vi "TypeConv_Register Existing Namespaces.vi"(10 "Existing Module":refnum<vi>, 11 "Namespaces":T1[](array[typedef])) -> ()   [LabVIEW 2013]
uses:
  Data Structures/JSON/Namespace.ctl
  Data Structures/JSON/Enum.ctl
  Data Structures/JSON/Enum Value.ctl
  Data Structures/JSON/Method.ctl
  Data Structures/JSON/Param.ctl
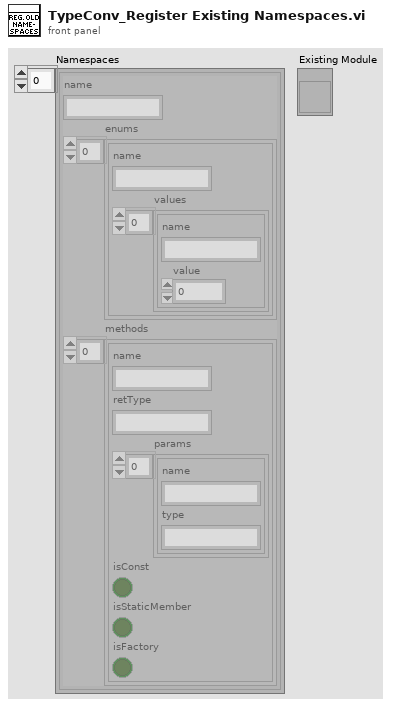
[diagram p1: front panel]
types:
  T1 = typedef "Namespace.ctl" = cluster{"name":string, "enums":T2[], "methods":T4[]}
  T2 = typedef "Enum.ctl" = cluster{"name":string, "values":T3[]}
  T3 = typedef "Enum Value.ctl" = cluster{"name":string, "value":i32}
  T4 = typedef "Method.ctl" = cluster{"name":string, "retType":string, "params":T5[], "isConst":bool, "isStaticMember":bool, "isFactory":bool}
  T5 = typedef "Param.ctl" = cluster{"name":string, "type":string}
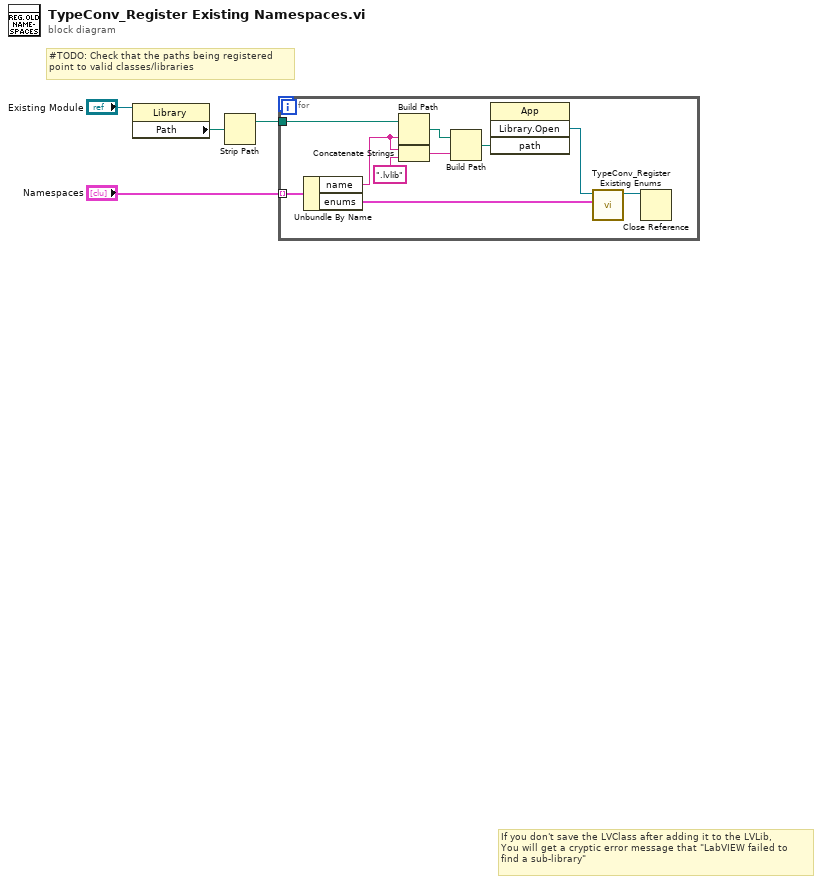
[diagram p0: block diagram]
diagram:
  # "#TODO: Check that the paths being registered\npoint to valid classes/libraries"
  # "If you don't save the LVClass after adding it to the LVLib,\nYou will get a cryptic error message that \"LabVIEW failed to\nfind a sub-library\""
  n1 = property class="Library"(reference="Existing Module") -> ("Path"=w2:path)  [unwired: 1 in, 2 out]
  n2 = Strip Path(path=w2) -> (stripped path=w1:path)  [unwired: 1 out]
  n3 = for {
    tunnel: "Namespaces" -> [w14] mode=indexing
    tunnel: w1 -> [w7]
    n4 = Unbundle By Name(w14) -> ("name"=w6:string, "enums"=w13:T2[])
    n5 = Build Path(base path=w7, name or relative path=w6) -> (appended path=w10:path)
    n6 = Concatenate Strings(w6, ".lvlib" ("string")) -> (w9:string)
    n7 = Build Path(base path=w10, name or relative path=w9) -> (appended path=w5:path)
    n8 = invoke class="App" method="Library.Open"("path"=w5) -> ("Open Library"=w12:refnum<vi>)  [unwired: 3 in, 3 out]
    n9 = call "TypeConv_Register Existing Enums.vi"("Enums"=w13, "Owning Lib"=w12) -> ("Owning Lib Dup"=w11:refnum<vi>)  [unwired: 9 in]
    n10 = Close Reference(reference=w11) -> ()  [unwired: 1 in, 1 out]
  }
